vi "capex AC power.vi"(3 "Enum":enum16{"2", "1"}(ring)) -> ()   [LabVIEW 2013]
panel:
  out "CV":bool
  out "CC":bool
  in  "stop":bool
  in  "Command power supply":bool
  out "Freq":dbl
  out "OCP":dbl
  out "OVP":dbl
  out "AC amps":dbl
  out "AC volts":dbl
  in  "AC Frequency":dbl
  in  "AC OCP":dbl
  in  "AC OVP":dbl
  in  "AC Amps":dbl
  in  "AC Voltage":dbl
  # "RMS volts"
  # "Amperes"
  # "Overvoltage protection limit"
  # "Overcurrent protection limit"
  # "Frequency"
  # "Actual"
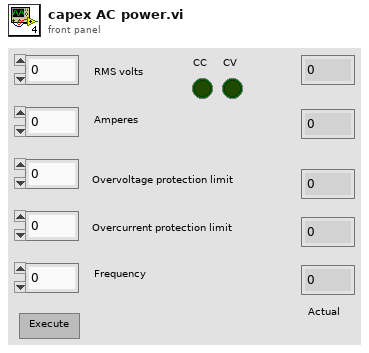
[diagram p1: front panel]
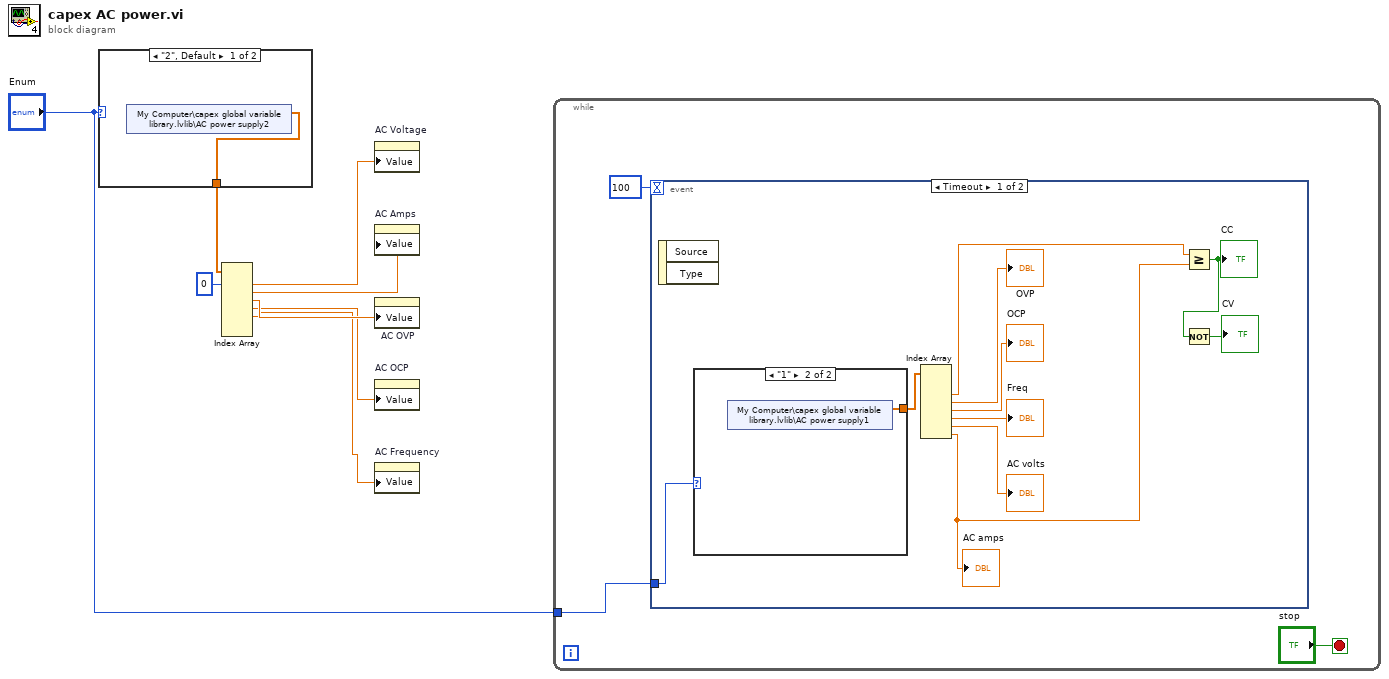
[diagram p0: block diagram]
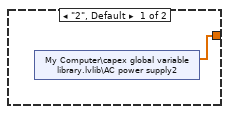
[diagram p2: hidden frame]
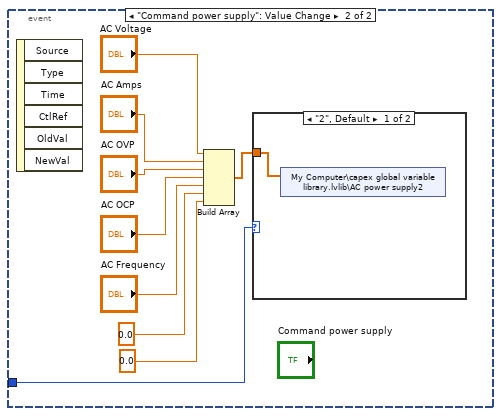
[diagram p3: hidden frame]
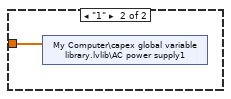
[diagram p4: hidden frame]
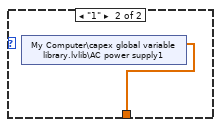
[diagram p5: hidden frame]
diagram:
  n1 = case shown="\"2\", Default" "Enum" {
    tunnel: [w9 w10] -> w2
    frame "2", Default {
      n2 = shared-variable "My Computer\\capex global variable library.lvlib\\AC power supply2"() -> (w9:dbl[])  [unwired: 1 in, 1 out]
    }
    frame "1" {
      n3 = shared-variable "My Computer\\capex global variable library.lvlib\\AC power supply1"() -> (w10:dbl[])  [unwired: 1 in, 1 out]
    }
  }
  n4 = Index Array(array=w2, index #1=0 ("index")) -> (element #1=w7:dbl, element #2=w6:dbl, element #3=w5:dbl, element #4=w4:dbl, element #5=w3:dbl)  [unwired: 6 in, 2 out]
  n5 = property on="AC Voltage" class="DigNum (strict)"("Value"=w7) -> ()  [unwired: 2 in, 2 out]
  n6 = property on="AC Amps" class="DigNum (strict)"("Value"=w6) -> ()  [unwired: 2 in, 2 out]
  n7 = property on="AC OVP" class="DigNum (strict)"("Value"=w5) -> ()  [unwired: 2 in, 2 out]
  n8 = property on="AC OCP" class="DigNum (strict)"("Value"=w4) -> ()  [unwired: 2 in, 2 out]
  n9 = property on="AC Frequency" class="DigNum (strict)"("Value"=w3) -> ()  [unwired: 2 in, 2 out]
  n10 = while {
    tunnel: "Enum" -> [w13]
    stop <- "stop" stop-if-true
    n11 = event shown="[0] Timeout" {
      selector: _ -> [_ _]
      dyn-events: _ -> [_ _]
      timeout: 100 -> [_ _]
      tunnel: w13 -> [w23 w34]
      event Timeout {
        n12 = event-data() -> ()  [unwired: 1 in, 2 out]
        n13 = case shown="\"1\"" w23 {
          tunnel: [w24 w25] -> w22
          frame "2", Default {
            n14 = shared-variable "My Computer\\capex global variable library.lvlib\\AC power supply2"() -> (w24:dbl[])  [unwired: 1 in, 1 out]
          }
          frame "1" {
            n15 = shared-variable "My Computer\\capex global variable library.lvlib\\AC power supply1"() -> (w25:dbl[])  [unwired: 1 in, 1 out]
          }
        }
        n16 = Index Array(array=w22) -> (element #2=w15:dbl, element #3=→"OVP":dbl, element #4=→"OCP":dbl, element #5=→"Freq":dbl, element #6=→"AC volts":dbl, element #7=w14:dbl)  [unwired: 7 in, 1 out]
        "AC amps" <- w14
        n17 = Greater Or Equal?(x=w15, y=w14) -> (x >= y?=w16:bool)
        "CC" <- w16
        n18 = Not(x=w16) -> (.not. x?=→"CV":bool)
      }
      event "Command power supply": Value Change {
        n19 = event-data() -> ()  [unwired: 1 in, 6 out]
        n20 = Build Array("AC Voltage", "AC Amps", "AC OVP", "AC OCP", "AC Frequency", 0.0 ("element"), 0.0 ("element")) -> (w28:dbl[])
        n21 = case shown="\"2\", Default" w34 {
          tunnel: w28 -> [w35 w36]
          frame "2", Default {
            n22 = shared-variable "My Computer\\capex global variable library.lvlib\\AC power supply2"(w35) -> ()  [unwired: 1 in, 1 out]
          }
          frame "1" {
            n23 = shared-variable "My Computer\\capex global variable library.lvlib\\AC power supply1"(w36) -> ()  [unwired: 1 in, 1 out]
          }
        }
      }
    }
  }
